vi "BASE.LoadConfig.vi"(8 "error in (no error)":errorcluster, 10 "config file path":path, 11 "Device.Simulation in":refnum<class "Device.Simulation.lvclass">) -> (0 "error out":errorcluster, 3 "Device.Simulation out":refnum<class "Device.Simulation.lvclass">)   [LabVIEW 2019, in "Device.Simulation.lvlib" / "Device.Simulation.lvclass"]
uses:
  Device.Simulation.lvclass
  Subsystems/BASE.Device/BASE.Device/BASE.Device.lvclass
  <vilib>/Utility/config.llb/NI_LVConfig.lvlib
panel:
  out "class name":string
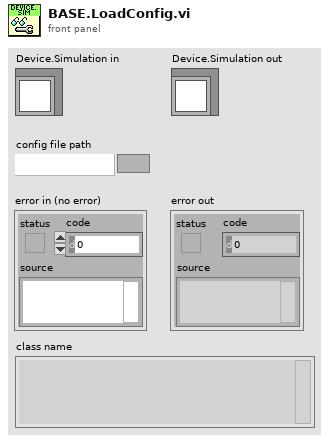
[diagram p1: front panel]
types:
  T1 = typedef "Device.Simulation.lvlib/Device.Simulation.lvclass/config--cluster.ctl" = cluster{"Name":string, "Time to Connect (ms)":u32, "Time to Check Connection (ms)":u32, "Time to Disconnect (ms)":u32, "Time to Read State (ms)":u32}
  T2 = typedef "NI_LVConfig.lvlib/Config Data RefNum.ctl" = refnum<k1>
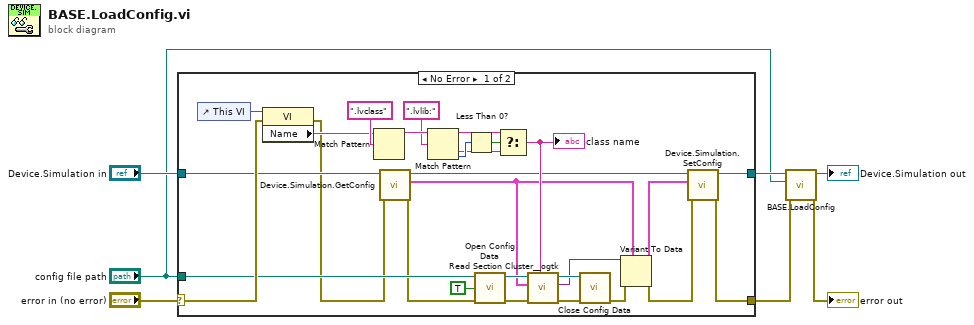
[diagram p0: block diagram]
diagram:
  n1 = case shown="No Error" "error in (no error)" {
    selector: "error in (no error)" -> [w29 w37]
    tunnel: [w9 w37] -> w4
    tunnel: [w15 w36] -> w3
    tunnel: "Device.Simulation in" -> [w14 w36]
    tunnel: "config file path" -> [w17 _]
    frame No Error {
      n2 = control-ref of="This VI"() -> (w31:refnum<vi>)
      n3 = property class="VI"(reference=w31, error in=w29) -> (error out=w11:errorcluster, "Name"=w18:string)  [unwired: 1 out]
      n4 = Match Pattern(string=w18, regular expression=".lvclass") -> (before substring=w25:string)  [unwired: 1 in, 3 out]
      n5 = call "Device.Simulation.GetConfig.vi"("error in (no error)"=w11, "Device.Simulation in"=w14) -> ("error out"=w8:errorcluster, "config"=w12:T1, "Device.Simulation out"=w13:refnum<class "Device.Simulation.lvclass">)  [unwired: 7 in]
      n6 = Match Pattern(string=w25, regular expression=".lvlib:") -> (before substring=w23:string, after substring=w22:string, offset past match=w26:i32)  [unwired: 1 in, 1 out]
      n7 = Less Than 0?(x=w26) -> (x < 0?=w24:bool)
      n8 = call <vilib>:"Open Config Data.vi"("error in (no error)"=w8, "create file if necessary (T)"=TRUE, "configuration file path"=w17) -> ("error out"=w34:errorcluster, "refnum"=w35:T2)  [unwired: 6 in, 1 out]
      n9 = Select(t=w23, s=w24, f=w22) -> (s? t:f=w19:string)
      "class name" <- w19
      n10 = call <userlib>:"Read Section Cluster__ogtk.vi"("section (optional)"=w19, "error in (no error)"=w34, "Section Formatted Cluster Type"=w12, "refnum"=w35) -> ("error out"=w33:errorcluster, "Section Formatted Cluster"=w28:variant, "dup refnum"=w32:T2)  [unwired: 3 in, 2 out]
      n11 = call <vilib>:"Close Config Data.vi"("error in (no error)"=w33, "refnum"=w32) -> ("error out"=w27:errorcluster)  [unwired: 8 in, 1 out]
      n12 = Variant To Data(error in=w27, type=w12, Variant=w28) -> (data=w16:T1, error out=w10:errorcluster)
      n13 = call "Device.Simulation.SetConfig.vi"("error in (no error)"=w10, "config"=w16, "Device.Simulation in"=w13) -> ("error out"=w9:errorcluster, "Device.Simulation out"=w15:refnum<class "Device.Simulation.lvclass">)  [unwired: 7 in]
    }
    frame Error {
    }
  }
  n14 = call-parent "BASE.LoadConfig.vi"("error in (no error)"=w4, "config file path"="config file path", "BASE.Device in"=w3) -> ("error out"=→"error out":errorcluster, "BASE.Device out"=→"Device.Simulation out":refnum<class "Device.Simulation.lvclass">)  [unwired: 7 in]
